vi "CanInstallStartup.vi"(4 "Version Selection (Highest)":u32(ring) items=["Highest", "Exactly"], 6 "Uninstall Conflicts (T)":bool=TRUE, 8 "error in (no error)":errorcluster, 10 "Startup Application":T1 {"component type" items=["standard", "hidden", "system", "unknown", "startup", "image"]}, 11 "Session in":refnum<k21>) -> (0 "error out":errorcluster, 1 "Broken Dependencies":T3[](array[typedef]) {"dependee"."component type" items=["standard", "hidden", "system", "unknown", "startup", "image"]; "depender"."component type" items=["standard", "hidden", "system", "unknown", "startup", "image"]}, 2 "Installing Components":T1[](array[typedef]) {"component type" items=["standard", "hidden", "system", "unknown", "startup", "image"]}, 3 "Session out":refnum<k21>, 5 "Uninstalling Components":T1[](array[typedef]) {"component type" items=["standard", "hidden", "system", "unknown", "startup", "image"]})   [LabVIEW 2014, in "nisyscfg.lvlib"]
uses:
  nisyscfg.lvlib
  Broken Dependency 1.2.ctl
  Software 1.2.ctl
  Component Type.ctl
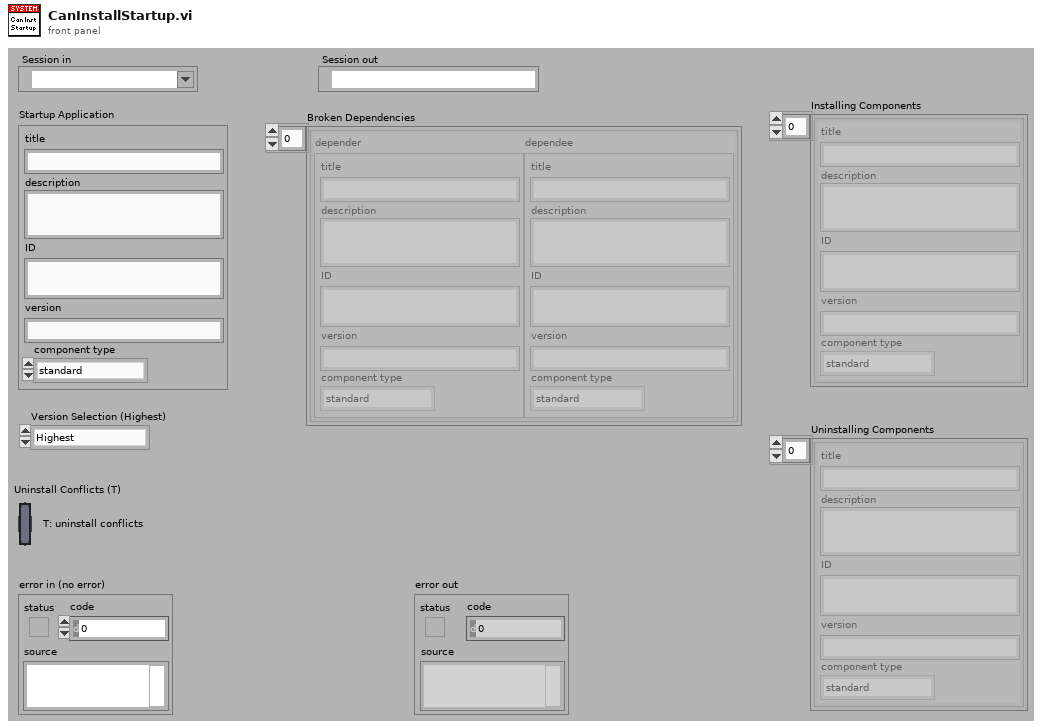
[diagram p1: front panel]
types:
  T1 = typedef "nisyscfg.lvlib/Software 1.2.ctl" = cluster{"title":string, "description":string, "ID":string, "version":string, "component type":T2}
  T2 = typedef "nisyscfg.lvlib/Component Type.ctl" = u32
  T3 = typedef "nisyscfg.lvlib/Broken Dependency 1.2.ctl" = cluster{"depender":T1, "dependee":T1}
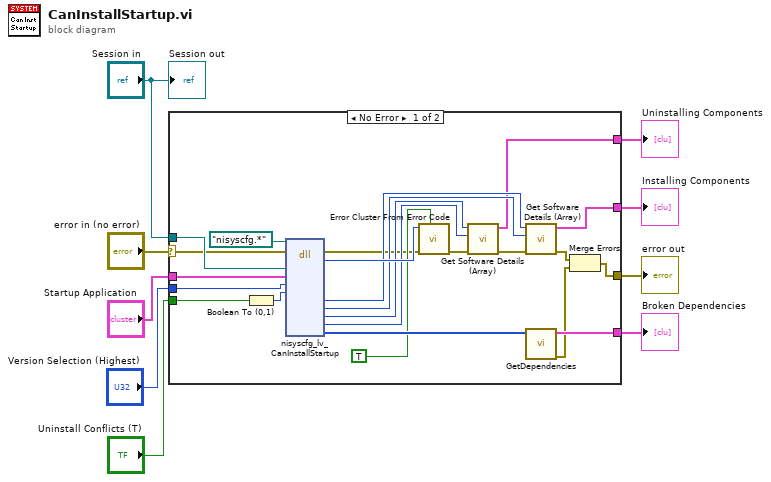
[diagram p0: block diagram]
diagram:
  n1 = case shown="No Error" "error in (no error)" {
    selector: "error in (no error)" -> [w25 w33]
    tunnel: "Session in" -> [w26 _]
    tunnel: [w27 w33] -> w4
    tunnel: [w30 _] -> w5
    tunnel: "Startup Application" -> [w23 _]
    tunnel: "Version Selection (Highest)" -> [w24 _]
    tunnel: "Uninstall Conflicts (T)" -> [w22 _]
    tunnel: [w16 _] -> w1
    tunnel: [w15 _] -> w2
    frame No Error {
      n2 = Boolean To (0,1)(Boolean=w22) -> (0, 1=w21:i16)
      n3 = dll-call lib="C:/projects/MAX/components/apis/trunk/5.0/objects/scs_nisyscfg_library_dynamic/win32U/i386/msvc90/debug/nisyscfg.dll" fn="nisyscfg_lv_CanInstallStartup" label="CanInstallStartup"(path in=path "nisyscfg.*", error in=w25, "session"=w26, "startupComponent"=w23, "versionSelectionMode"=w24, "uninstallConflicts"=w21) -> (error out=w10:errorcluster, "result"=w32:i32, "installingComponents"=w20:u64, "installingCount"=w19:i32, "uninstallingComponents"=w18:u64, "uninstallingCount"=w17:i32, "brokenDependencies"=w31:u64[])  [unwired: 10 in, 1 out]
      n4 = call "Error Cluster From Error Code.vi"("show call chain? (False)"=TRUE, "error in (no error)"=w10, "error code (0)"=w32) -> ("error out"=w11:errorcluster)  [unwired: 6 in]
      n5 = call "Get Software Details (Array).vi"("error in (no error)"=w11, "Number of Elements"=w17, "Enumerator in"=w18) -> ("error out"=w14:errorcluster, "Software Components"=w15:T1[])  [unwired: 7 in]
      n6 = call "Get Software Details (Array).vi"("error in (no error)"=w14, "Number of Elements"=w19, "Enumerator in"=w20) -> ("error out"=w12:errorcluster, "Software Components"=w16:T1[])  [unwired: 7 in]
      n7 = call "GetDependencies.vi"("Enumerator in"=w31) -> ("error out"=w13:errorcluster, "Dependencies"=w30:T3[])  [unwired: 9 in]
      n8 = Merge Errors(w12, w13) -> (w27:errorcluster)
    }
    frame Error {
    }
  }
  "error out" <- w4
  "Broken Dependencies" <- w5
  "Installing Components" <- w1
  "Uninstalling Components" <- w2
  "Session out" <- "Session in"
